vi "switch_data_process_switch-status.vi"() -> (0 "Switch_V_R":dbl[][](array[numeric]), 1 "Switch_V_L":dbl[][](array[numeric]), 2 "switch_FREQ_R":dbl[](array[numeric]), 3 "switch_FREQ_L":dbl[](array[numeric]), 4 "switch_RPF":dbl[](array[numeric]), 5 "switch_APF":dbl[](array[numeric]), 6 "switch_status":bool[](array[boolean]))   [LabVIEW 2016]
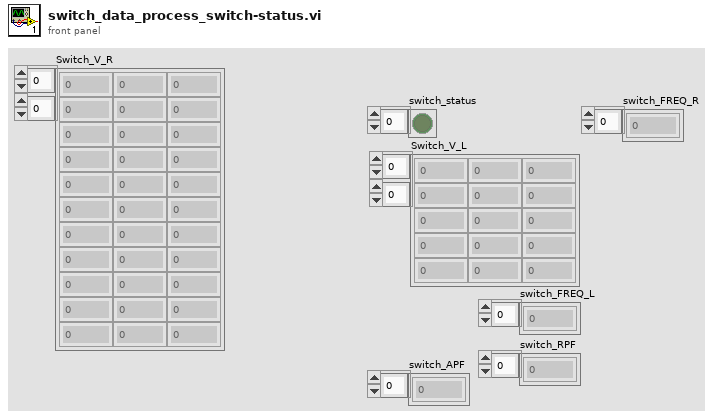
[diagram p1: front panel]
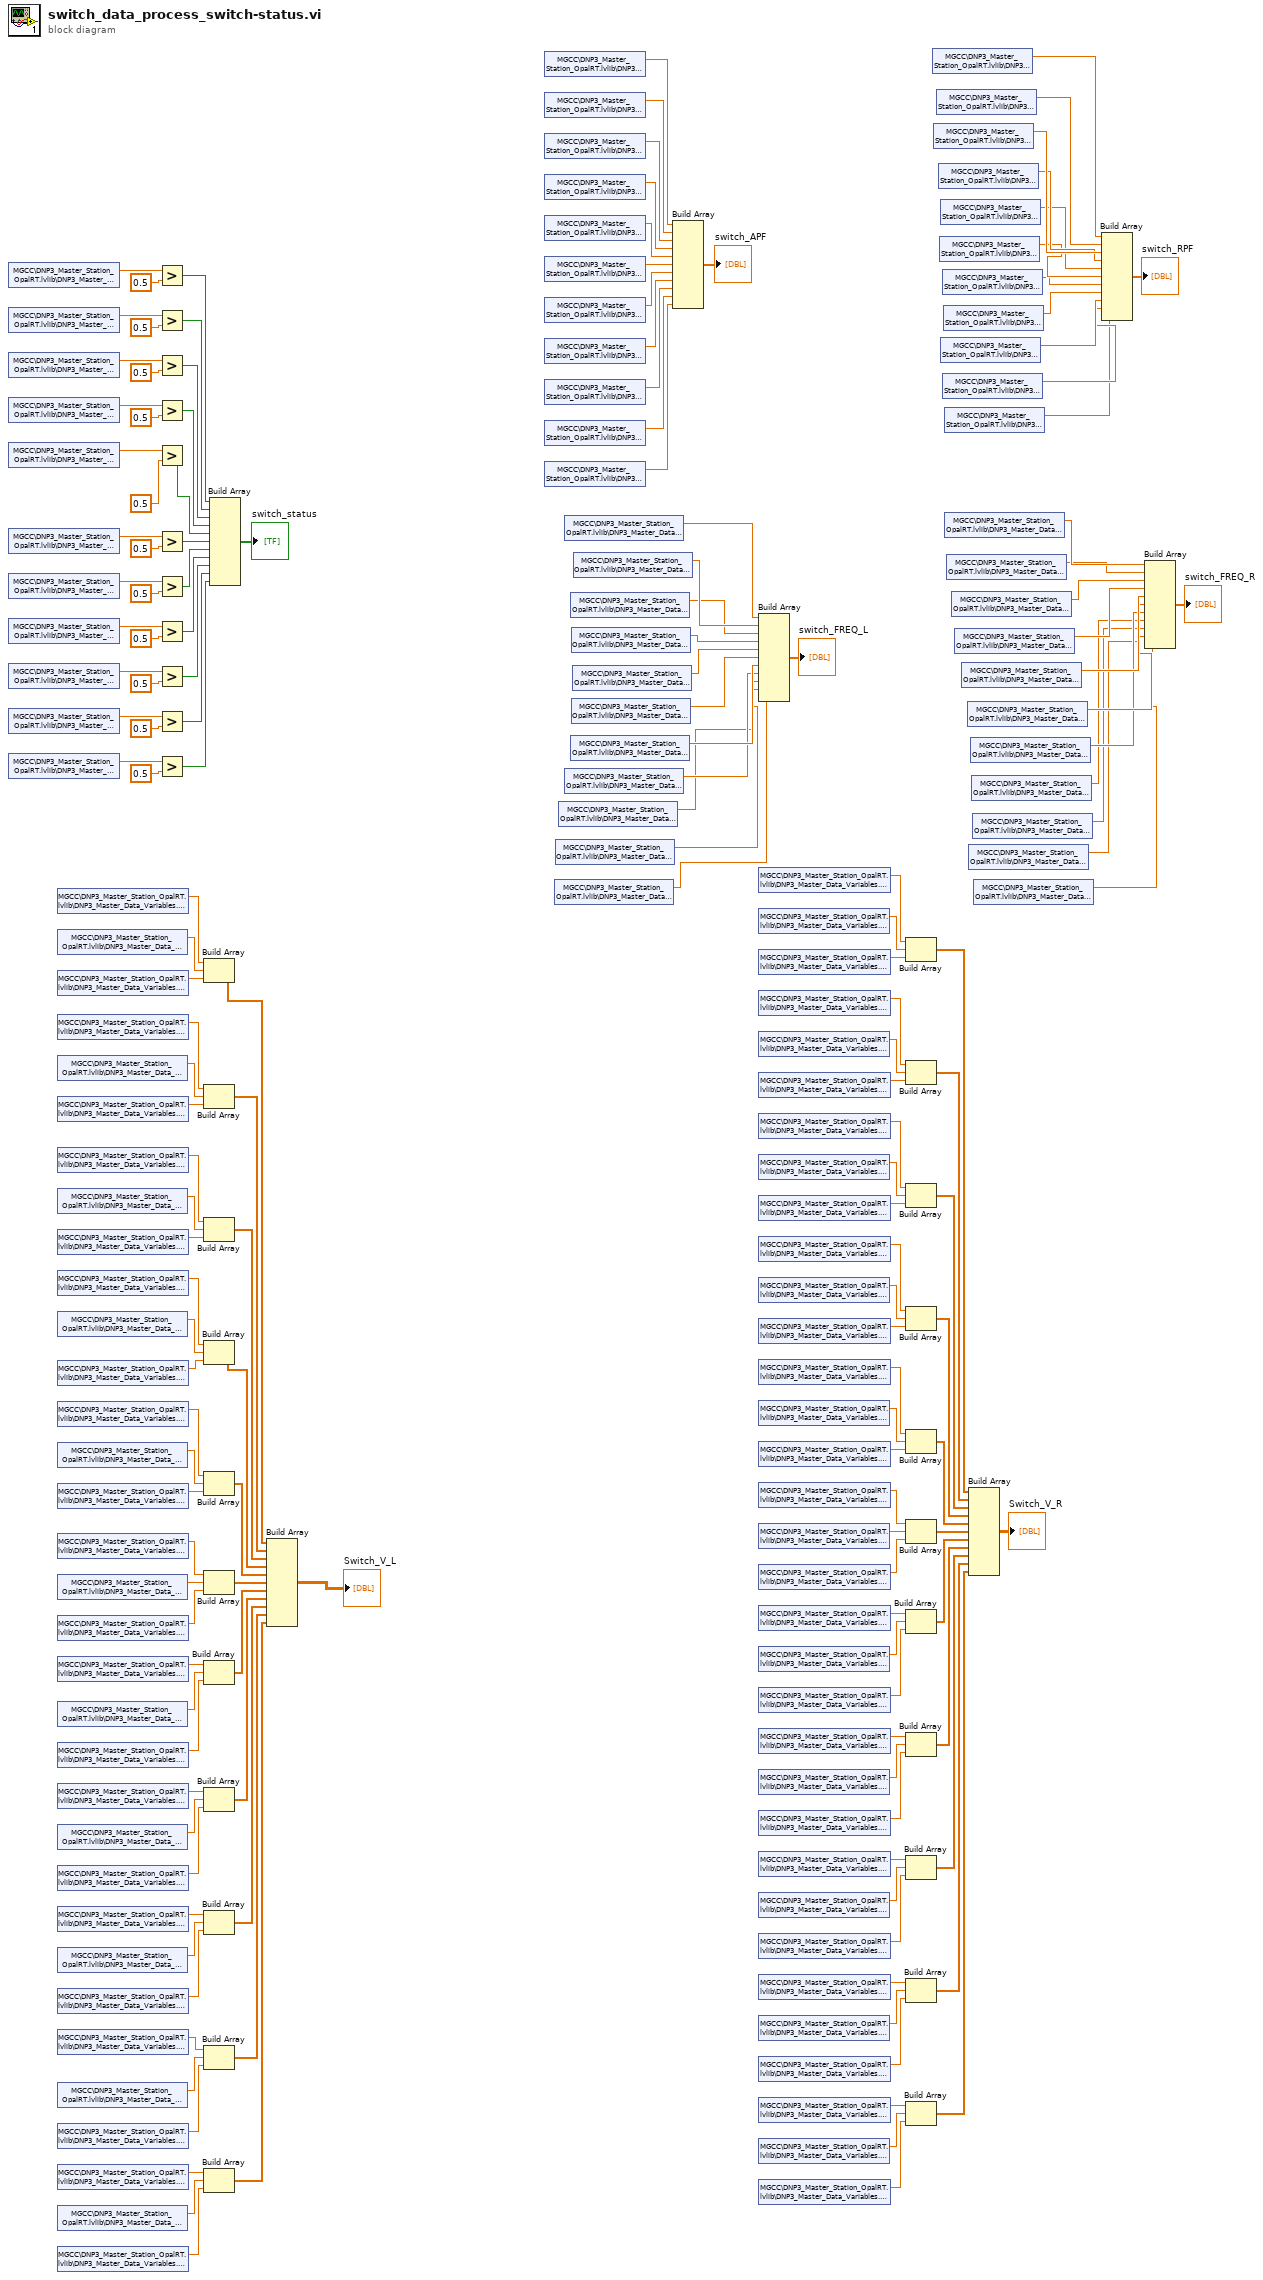
[diagram p0: block diagram]
diagram:
  n1 = shared-variable "MGCC\\DNP3_Master_Station_OpalRT.lvlib\\DNP3_Master_Data_Variables.lvlib\\MS_Analog_Status.lvlib\\S0102-status"() -> (w170:dbl)  [unwired: 1 in, 1 out]
  n2 = shared-variable "MGCC\\DNP3_Master_Station_OpalRT.lvlib\\DNP3_Master_Data_Variables.lvlib\\MS_Analog_Status.lvlib\\S0203-status"() -> (w159:dbl)  [unwired: 1 in, 1 out]
  n3 = shared-variable "MGCC\\DNP3_Master_Station_OpalRT.lvlib\\DNP3_Master_Data_Variables.lvlib\\MS_Analog_Status.lvlib\\S0304-status"() -> (w158:dbl)  [unwired: 1 in, 1 out]
  n4 = shared-variable "MGCC\\DNP3_Master_Station_OpalRT.lvlib\\DNP3_Master_Data_Variables.lvlib\\MS_Analog_Status.lvlib\\S0307-status"() -> (w157:dbl)  [unwired: 1 in, 1 out]
  n5 = shared-variable "MGCC\\DNP3_Master_Station_OpalRT.lvlib\\DNP3_Master_Data_Variables.lvlib\\MS_Analog_Status.lvlib\\S0405-status"() -> (w156:dbl)  [unwired: 1 in, 1 out]
  n6 = shared-variable "MGCC\\DNP3_Master_Station_OpalRT.lvlib\\DNP3_Master_Data_Variables.lvlib\\MS_Analog_Status.lvlib\\S0406-status"() -> (w155:dbl)  [unwired: 1 in, 1 out]
  n7 = shared-variable "MGCC\\DNP3_Master_Station_OpalRT.lvlib\\DNP3_Master_Data_Variables.lvlib\\MS_Analog_Status.lvlib\\S0708-status"() -> (w154:dbl)  [unwired: 1 in, 1 out]
  n8 = shared-variable "MGCC\\DNP3_Master_Station_OpalRT.lvlib\\DNP3_Master_Data_Variables.lvlib\\MS_Analog_Status.lvlib\\S0709-status"() -> (w153:dbl)  [unwired: 1 in, 1 out]
  n9 = shared-variable "MGCC\\DNP3_Master_Station_OpalRT.lvlib\\DNP3_Master_Data_Variables.lvlib\\MS_Analog_Status.lvlib\\S0910-status"() -> (w152:dbl)  [unwired: 1 in, 1 out]
  n10 = shared-variable "MGCC\\DNP3_Master_Station_OpalRT.lvlib\\DNP3_Master_Data_Variables.lvlib\\MS_Analog_Status.lvlib\\S1011-status"() -> (w151:dbl)  [unwired: 1 in, 1 out]
  n11 = shared-variable "MGCC\\DNP3_Master_Station_OpalRT.lvlib\\DNP3_Master_Data_Variables.lvlib\\MS_Analog_Status.lvlib\\S1114-status"() -> (w150:dbl)  [unwired: 1 in, 1 out]
  n12 = shared-variable "MGCC\\DNP3_Master_Station_OpalRT.lvlib\\DNP3_Master_Data_Variables.lvlib\\MS_Analog_Status.lvlib\\S0102-MAG-A-L"() -> (w138:dbl)  [unwired: 1 in, 1 out]
  n13 = shared-variable "MGCC\\DNP3_Master_Station_OpalRT.lvlib\\DNP3_Master_Data_Variables.lvlib\\MS_Analog_Status.lvlib\\S0102-MAG-B-L"() -> (w137:dbl)  [unwired: 1 in, 1 out]
  n14 = shared-variable "MGCC\\DNP3_Master_Station_OpalRT.lvlib\\DNP3_Master_Data_Variables.lvlib\\MS_Analog_Status.lvlib\\S0102-MAG-C-L"() -> (w136:dbl)  [unwired: 1 in, 1 out]
  n15 = shared-variable "MGCC\\DNP3_Master_Station_OpalRT.lvlib\\DNP3_Master_Data_Variables.lvlib\\MS_Analog_Status.lvlib\\S0203-MAG-A-L"() -> (w127:dbl)  [unwired: 1 in, 1 out]
  n16 = shared-variable "MGCC\\DNP3_Master_Station_OpalRT.lvlib\\DNP3_Master_Data_Variables.lvlib\\MS_Analog_Status.lvlib\\S0203-MAG-B-L"() -> (w126:dbl)  [unwired: 1 in, 1 out]
  n17 = shared-variable "MGCC\\DNP3_Master_Station_OpalRT.lvlib\\DNP3_Master_Data_Variables.lvlib\\MS_Analog_Status.lvlib\\S0203-MAG-C-L"() -> (w125:dbl)  [unwired: 1 in, 1 out]
  n18 = shared-variable "MGCC\\DNP3_Master_Station_OpalRT.lvlib\\DNP3_Master_Data_Variables.lvlib\\MS_Analog_Status.lvlib\\S0304-MAG-A-L"() -> (w122:dbl)  [unwired: 1 in, 1 out]
  n19 = shared-variable "MGCC\\DNP3_Master_Station_OpalRT.lvlib\\DNP3_Master_Data_Variables.lvlib\\MS_Analog_Status.lvlib\\S0304-MAG-B-L"() -> (w121:dbl)  [unwired: 1 in, 1 out]
  n20 = shared-variable "MGCC\\DNP3_Master_Station_OpalRT.lvlib\\DNP3_Master_Data_Variables.lvlib\\MS_Analog_Status.lvlib\\S0304-MAG-C-L"() -> (w120:dbl)  [unwired: 1 in, 1 out]
  n21 = shared-variable "MGCC\\DNP3_Master_Station_OpalRT.lvlib\\DNP3_Master_Data_Variables.lvlib\\MS_Analog_Status.lvlib\\S0307-MAG-A-L"() -> (w118:dbl)  [unwired: 1 in, 1 out]
  n22 = shared-variable "MGCC\\DNP3_Master_Station_OpalRT.lvlib\\DNP3_Master_Data_Variables.lvlib\\MS_Analog_Status.lvlib\\S0307-MAG-B-L"() -> (w117:dbl)  [unwired: 1 in, 1 out]
  n23 = shared-variable "MGCC\\DNP3_Master_Station_OpalRT.lvlib\\DNP3_Master_Data_Variables.lvlib\\MS_Analog_Status.lvlib\\S0307-MAG-C-L"() -> (w116:dbl)  [unwired: 1 in, 1 out]
  n24 = shared-variable "MGCC\\DNP3_Master_Station_OpalRT.lvlib\\DNP3_Master_Data_Variables.lvlib\\MS_Analog_Status.lvlib\\S0405-MAG-A-L"() -> (w114:dbl)  [unwired: 1 in, 1 out]
  n25 = shared-variable "MGCC\\DNP3_Master_Station_OpalRT.lvlib\\DNP3_Master_Data_Variables.lvlib\\MS_Analog_Status.lvlib\\S0405-MAG-B-L"() -> (w113:dbl)  [unwired: 1 in, 1 out]
  n26 = shared-variable "MGCC\\DNP3_Master_Station_OpalRT.lvlib\\DNP3_Master_Data_Variables.lvlib\\MS_Analog_Status.lvlib\\S0405-MAG-C-L"() -> (w112:dbl)  [unwired: 1 in, 1 out]
  n27 = shared-variable "MGCC\\DNP3_Master_Station_OpalRT.lvlib\\DNP3_Master_Data_Variables.lvlib\\MS_Analog_Status.lvlib\\S0406-MAG-A-L"() -> (w110:dbl)  [unwired: 1 in, 1 out]
  n28 = shared-variable "MGCC\\DNP3_Master_Station_OpalRT.lvlib\\DNP3_Master_Data_Variables.lvlib\\MS_Analog_Status.lvlib\\S0406-MAG-B-L"() -> (w109:dbl)  [unwired: 1 in, 1 out]
  n29 = shared-variable "MGCC\\DNP3_Master_Station_OpalRT.lvlib\\DNP3_Master_Data_Variables.lvlib\\MS_Analog_Status.lvlib\\S0406-MAG-C-L"() -> (w108:dbl)  [unwired: 1 in, 1 out]
  n30 = shared-variable "MGCC\\DNP3_Master_Station_OpalRT.lvlib\\DNP3_Master_Data_Variables.lvlib\\MS_Analog_Status.lvlib\\S0708-MAG-A-L"() -> (w106:dbl)  [unwired: 1 in, 1 out]
  n31 = shared-variable "MGCC\\DNP3_Master_Station_OpalRT.lvlib\\DNP3_Master_Data_Variables.lvlib\\MS_Analog_Status.lvlib\\S0708-MAG-B-L"() -> (w105:dbl)  [unwired: 1 in, 1 out]
  n32 = shared-variable "MGCC\\DNP3_Master_Station_OpalRT.lvlib\\DNP3_Master_Data_Variables.lvlib\\MS_Analog_Status.lvlib\\S0708-MAG-C-L"() -> (w104:dbl)  [unwired: 1 in, 1 out]
  n33 = shared-variable "MGCC\\DNP3_Master_Station_OpalRT.lvlib\\DNP3_Master_Data_Variables.lvlib\\MS_Analog_Status.lvlib\\S0709-MAG-A-L"() -> (w102:dbl)  [unwired: 1 in, 1 out]
  n34 = shared-variable "MGCC\\DNP3_Master_Station_OpalRT.lvlib\\DNP3_Master_Data_Variables.lvlib\\MS_Analog_Status.lvlib\\S0709-MAG-B-L"() -> (w101:dbl)  [unwired: 1 in, 1 out]
  n35 = shared-variable "MGCC\\DNP3_Master_Station_OpalRT.lvlib\\DNP3_Master_Data_Variables.lvlib\\MS_Analog_Status.lvlib\\S0709-MAG-C-L"() -> (w100:dbl)  [unwired: 1 in, 1 out]
  n36 = shared-variable "MGCC\\DNP3_Master_Station_OpalRT.lvlib\\DNP3_Master_Data_Variables.lvlib\\MS_Analog_Status.lvlib\\S0910-MAG-A-L"() -> (w98:dbl)  [unwired: 1 in, 1 out]
  n37 = shared-variable "MGCC\\DNP3_Master_Station_OpalRT.lvlib\\DNP3_Master_Data_Variables.lvlib\\MS_Analog_Status.lvlib\\S0910-MAG-B-L"() -> (w97:dbl)  [unwired: 1 in, 1 out]
  n38 = shared-variable "MGCC\\DNP3_Master_Station_OpalRT.lvlib\\DNP3_Master_Data_Variables.lvlib\\MS_Analog_Status.lvlib\\S0910-MAG-C-L"() -> (w96:dbl)  [unwired: 1 in, 1 out]
  n39 = shared-variable "MGCC\\DNP3_Master_Station_OpalRT.lvlib\\DNP3_Master_Data_Variables.lvlib\\MS_Analog_Status.lvlib\\S1011-MAG-A-L"() -> (w94:dbl)  [unwired: 1 in, 1 out]
  n40 = shared-variable "MGCC\\DNP3_Master_Station_OpalRT.lvlib\\DNP3_Master_Data_Variables.lvlib\\MS_Analog_Status.lvlib\\S1011-MAG-B-L"() -> (w93:dbl)  [unwired: 1 in, 1 out]
  n41 = shared-variable "MGCC\\DNP3_Master_Station_OpalRT.lvlib\\DNP3_Master_Data_Variables.lvlib\\MS_Analog_Status.lvlib\\S1011-MAG-C-L"() -> (w92:dbl)  [unwired: 1 in, 1 out]
  n42 = shared-variable "MGCC\\DNP3_Master_Station_OpalRT.lvlib\\DNP3_Master_Data_Variables.lvlib\\MS_Analog_Status.lvlib\\S1114-MAG-A-L"() -> (w90:dbl)  [unwired: 1 in, 1 out]
  n43 = shared-variable "MGCC\\DNP3_Master_Station_OpalRT.lvlib\\DNP3_Master_Data_Variables.lvlib\\MS_Analog_Status.lvlib\\S1114-MAG-B-L"() -> (w89:dbl)  [unwired: 1 in, 1 out]
  n44 = shared-variable "MGCC\\DNP3_Master_Station_OpalRT.lvlib\\DNP3_Master_Data_Variables.lvlib\\MS_Analog_Status.lvlib\\S1114-MAG-C-L"() -> (w88:dbl)  [unwired: 1 in, 1 out]
  n45 = Greater?(x=w170, y=0.5) -> (0:w171:bool)
  n46 = Greater?(x=w159, y=0.5) -> (0:w149:bool)
  n47 = Greater?(x=w158, y=0.5) -> (0:w148:bool)
  n48 = Greater?(x=w157, y=0.5) -> (0:w147:bool)
  n49 = Greater?(x=w156, y=0.5) -> (0:w146:bool)
  n50 = Greater?(x=w155, y=0.5) -> (0:w145:bool)
  n51 = Greater?(x=w154, y=0.5) -> (0:w144:bool)
  n52 = Greater?(x=w153, y=0.5) -> (0:w143:bool)
  n53 = Greater?(x=w152, y=0.5) -> (0:w142:bool)
  n54 = Greater?(x=w151, y=0.5) -> (0:w141:bool)
  n55 = Greater?(x=w150, y=0.5) -> (0:w140:bool)
  n56 = Build Array(w138, w137, w136) -> (w135:dbl[])
  n57 = Build Array(w127, w126, w125) -> (w124:dbl[])
  n58 = Build Array(w122, w121, w120) -> (w119:dbl[])
  n59 = Build Array(w118, w117, w116) -> (w115:dbl[])
  n60 = Build Array(w114, w113, w112) -> (w111:dbl[])
  n61 = Build Array(w110, w109, w108) -> (w107:dbl[])
  n62 = Build Array(w106, w105, w104) -> (w103:dbl[])
  n63 = Build Array(w102, w101, w100) -> (w99:dbl[])
  n64 = Build Array(w98, w97, w96) -> (w95:dbl[])
  n65 = Build Array(w94, w93, w92) -> (w91:dbl[])
  n66 = Build Array(w90, w89, w88) -> (w87:dbl[])
  n67 = Build Array(w171, w149, w148, w147, w146, w145, w144, w143, w142, w141, w140) -> (→"switch_status":bool[])
  n68 = Build Array(w135, w124, w119, w115, w111, w107, w103, w99, w95, w91, w87) -> (→"Switch_V_L":dbl[][])
  n69 = shared-variable "MGCC\\DNP3_Master_Station_OpalRT.lvlib\\DNP3_Master_Data_Variables.lvlib\\MS_Analog_Status.lvlib\\S0102-APF"() -> (w48:dbl)  [unwired: 1 in, 1 out]
  n70 = shared-variable "MGCC\\DNP3_Master_Station_OpalRT.lvlib\\DNP3_Master_Data_Variables.lvlib\\MS_Analog_Status.lvlib\\S0203-APF"() -> (w47:dbl)  [unwired: 1 in, 1 out]
  n71 = shared-variable "MGCC\\DNP3_Master_Station_OpalRT.lvlib\\DNP3_Master_Data_Variables.lvlib\\MS_Analog_Status.lvlib\\S0304-APF"() -> (w46:dbl)  [unwired: 1 in, 1 out]
  n72 = shared-variable "MGCC\\DNP3_Master_Station_OpalRT.lvlib\\DNP3_Master_Data_Variables.lvlib\\MS_Analog_Status.lvlib\\S0307-APF"() -> (w45:dbl)  [unwired: 1 in, 1 out]
  n73 = shared-variable "MGCC\\DNP3_Master_Station_OpalRT.lvlib\\DNP3_Master_Data_Variables.lvlib\\MS_Analog_Status.lvlib\\S0405-APF"() -> (w44:dbl)  [unwired: 1 in, 1 out]
  n74 = shared-variable "MGCC\\DNP3_Master_Station_OpalRT.lvlib\\DNP3_Master_Data_Variables.lvlib\\MS_Analog_Status.lvlib\\S0406-APF"() -> (w43:dbl)  [unwired: 1 in, 1 out]
  n75 = shared-variable "MGCC\\DNP3_Master_Station_OpalRT.lvlib\\DNP3_Master_Data_Variables.lvlib\\MS_Analog_Status.lvlib\\S0708-APF"() -> (w42:dbl)  [unwired: 1 in, 1 out]
  n76 = shared-variable "MGCC\\DNP3_Master_Station_OpalRT.lvlib\\DNP3_Master_Data_Variables.lvlib\\MS_Analog_Status.lvlib\\S0709-APF"() -> (w41:dbl)  [unwired: 1 in, 1 out]
  n77 = shared-variable "MGCC\\DNP3_Master_Station_OpalRT.lvlib\\DNP3_Master_Data_Variables.lvlib\\MS_Analog_Status.lvlib\\S0910-APF"() -> (w40:dbl)  [unwired: 1 in, 1 out]
  n78 = shared-variable "MGCC\\DNP3_Master_Station_OpalRT.lvlib\\DNP3_Master_Data_Variables.lvlib\\MS_Analog_Status.lvlib\\S1011-APF"() -> (w39:dbl)  [unwired: 1 in, 1 out]
  n79 = shared-variable "MGCC\\DNP3_Master_Station_OpalRT.lvlib\\DNP3_Master_Data_Variables.lvlib\\MS_Analog_Status.lvlib\\S1114-APF"() -> (w38:dbl)  [unwired: 1 in, 1 out]
  n80 = shared-variable "MGCC\\DNP3_Master_Station_OpalRT.lvlib\\DNP3_Master_Data_Variables.lvlib\\MS_Analog_Status.lvlib\\S1114-FREQ-L"() -> (w26:dbl)  [unwired: 1 in, 1 out]
  n81 = shared-variable "MGCC\\DNP3_Master_Station_OpalRT.lvlib\\DNP3_Master_Data_Variables.lvlib\\MS_Analog_Status.lvlib\\S1011-FREQ-L"() -> (w27:dbl)  [unwired: 1 in, 1 out]
  n82 = shared-variable "MGCC\\DNP3_Master_Station_OpalRT.lvlib\\DNP3_Master_Data_Variables.lvlib\\MS_Analog_Status.lvlib\\S0910-FREQ-L"() -> (w28:dbl)  [unwired: 1 in, 1 out]
  n83 = shared-variable "MGCC\\DNP3_Master_Station_OpalRT.lvlib\\DNP3_Master_Data_Variables.lvlib\\MS_Analog_Status.lvlib\\S0102-FREQ-L"() -> (w36:dbl)  [unwired: 1 in, 1 out]
  n84 = shared-variable "MGCC\\DNP3_Master_Station_OpalRT.lvlib\\DNP3_Master_Data_Variables.lvlib\\MS_Analog_Status.lvlib\\S0709-FREQ-L"() -> (w29:dbl)  [unwired: 1 in, 1 out]
  n85 = shared-variable "MGCC\\DNP3_Master_Station_OpalRT.lvlib\\DNP3_Master_Data_Variables.lvlib\\MS_Analog_Status.lvlib\\S0304-FREQ-L"() -> (w34:dbl)  [unwired: 1 in, 1 out]
  n86 = shared-variable "MGCC\\DNP3_Master_Station_OpalRT.lvlib\\DNP3_Master_Data_Variables.lvlib\\MS_Analog_Status.lvlib\\S0708-FREQ-L"() -> (w30:dbl)  [unwired: 1 in, 1 out]
  n87 = shared-variable "MGCC\\DNP3_Master_Station_OpalRT.lvlib\\DNP3_Master_Data_Variables.lvlib\\MS_Analog_Status.lvlib\\S0307-FREQ-L"() -> (w33:dbl)  [unwired: 1 in, 1 out]
  n88 = shared-variable "MGCC\\DNP3_Master_Station_OpalRT.lvlib\\DNP3_Master_Data_Variables.lvlib\\MS_Analog_Status.lvlib\\S0406-FREQ-L"() -> (w31:dbl)  [unwired: 1 in, 1 out]
  n89 = shared-variable "MGCC\\DNP3_Master_Station_OpalRT.lvlib\\DNP3_Master_Data_Variables.lvlib\\MS_Analog_Status.lvlib\\S0405-FREQ-L"() -> (w32:dbl)  [unwired: 1 in, 1 out]
  n90 = shared-variable "MGCC\\DNP3_Master_Station_OpalRT.lvlib\\DNP3_Master_Data_Variables.lvlib\\MS_Analog_Status.lvlib\\S0203-FREQ-L"() -> (w35:dbl)  [unwired: 1 in, 1 out]
  n91 = Build Array(w48, w47, w46, w45, w44, w43, w42, w41, w40, w39, w38) -> (→"switch_APF":dbl[])
  n92 = Build Array(w36, w35, w34, w33, w32, w31, w30, w29, w28, w27, w26) -> (→"switch_FREQ_L":dbl[])
  n93 = shared-variable "MGCC\\DNP3_Master_Station_OpalRT.lvlib\\DNP3_Master_Data_Variables.lvlib\\MS_Analog_Status.lvlib\\S0102-MAG-A-R"() -> (w134:dbl)  [unwired: 1 in, 1 out]
  n94 = shared-variable "MGCC\\DNP3_Master_Station_OpalRT.lvlib\\DNP3_Master_Data_Variables.lvlib\\MS_Analog_Status.lvlib\\S0102-MAG-B-R"() -> (w133:dbl)  [unwired: 1 in, 1 out]
  n95 = shared-variable "MGCC\\DNP3_Master_Station_OpalRT.lvlib\\DNP3_Master_Data_Variables.lvlib\\MS_Analog_Status.lvlib\\S0102-MAG-C-R"() -> (w132:dbl)  [unwired: 1 in, 1 out]
  n96 = shared-variable "MGCC\\DNP3_Master_Station_OpalRT.lvlib\\DNP3_Master_Data_Variables.lvlib\\MS_Analog_Status.lvlib\\S0203-MAG-A-R"() -> (w130:dbl)  [unwired: 1 in, 1 out]
  n97 = shared-variable "MGCC\\DNP3_Master_Station_OpalRT.lvlib\\DNP3_Master_Data_Variables.lvlib\\MS_Analog_Status.lvlib\\S0203-MAG-B-R"() -> (w129:dbl)  [unwired: 1 in, 1 out]
  n98 = shared-variable "MGCC\\DNP3_Master_Station_OpalRT.lvlib\\DNP3_Master_Data_Variables.lvlib\\MS_Analog_Status.lvlib\\S0203-MAG-C-R"() -> (w128:dbl)  [unwired: 1 in, 1 out]
  n99 = shared-variable "MGCC\\DNP3_Master_Station_OpalRT.lvlib\\DNP3_Master_Data_Variables.lvlib\\MS_Analog_Status.lvlib\\S0304-MAG-A-R"() -> (w86:dbl)  [unwired: 1 in, 1 out]
  n100 = shared-variable "MGCC\\DNP3_Master_Station_OpalRT.lvlib\\DNP3_Master_Data_Variables.lvlib\\MS_Analog_Status.lvlib\\S0304-MAG-B-R"() -> (w85:dbl)  [unwired: 1 in, 1 out]
  n101 = shared-variable "MGCC\\DNP3_Master_Station_OpalRT.lvlib\\DNP3_Master_Data_Variables.lvlib\\MS_Analog_Status.lvlib\\S0304-MAG-C-R"() -> (w84:dbl)  [unwired: 1 in, 1 out]
  n102 = shared-variable "MGCC\\DNP3_Master_Station_OpalRT.lvlib\\DNP3_Master_Data_Variables.lvlib\\MS_Analog_Status.lvlib\\S0307-MAG-A-R"() -> (w82:dbl)  [unwired: 1 in, 1 out]
  n103 = shared-variable "MGCC\\DNP3_Master_Station_OpalRT.lvlib\\DNP3_Master_Data_Variables.lvlib\\MS_Analog_Status.lvlib\\S0307-MAG-B-R"() -> (w81:dbl)  [unwired: 1 in, 1 out]
  n104 = shared-variable "MGCC\\DNP3_Master_Station_OpalRT.lvlib\\DNP3_Master_Data_Variables.lvlib\\MS_Analog_Status.lvlib\\S0307-MAG-C-R"() -> (w80:dbl)  [unwired: 1 in, 1 out]
  n105 = shared-variable "MGCC\\DNP3_Master_Station_OpalRT.lvlib\\DNP3_Master_Data_Variables.lvlib\\MS_Analog_Status.lvlib\\S0405-MAG-A-R"() -> (w78:dbl)  [unwired: 1 in, 1 out]
  n106 = shared-variable "MGCC\\DNP3_Master_Station_OpalRT.lvlib\\DNP3_Master_Data_Variables.lvlib\\MS_Analog_Status.lvlib\\S0405-MAG-B-R"() -> (w77:dbl)  [unwired: 1 in, 1 out]
  n107 = shared-variable "MGCC\\DNP3_Master_Station_OpalRT.lvlib\\DNP3_Master_Data_Variables.lvlib\\MS_Analog_Status.lvlib\\S0405-MAG-C-R"() -> (w76:dbl)  [unwired: 1 in, 1 out]
  n108 = shared-variable "MGCC\\DNP3_Master_Station_OpalRT.lvlib\\DNP3_Master_Data_Variables.lvlib\\MS_Analog_Status.lvlib\\S0406-MAG-A-R"() -> (w74:dbl)  [unwired: 1 in, 1 out]
  n109 = shared-variable "MGCC\\DNP3_Master_Station_OpalRT.lvlib\\DNP3_Master_Data_Variables.lvlib\\MS_Analog_Status.lvlib\\S0406-MAG-B-R"() -> (w73:dbl)  [unwired: 1 in, 1 out]
  n110 = shared-variable "MGCC\\DNP3_Master_Station_OpalRT.lvlib\\DNP3_Master_Data_Variables.lvlib\\MS_Analog_Status.lvlib\\S0406-MAG-C-R"() -> (w72:dbl)  [unwired: 1 in, 1 out]
  n111 = shared-variable "MGCC\\DNP3_Master_Station_OpalRT.lvlib\\DNP3_Master_Data_Variables.lvlib\\MS_Analog_Status.lvlib\\S0708-MAG-A-R"() -> (w70:dbl)  [unwired: 1 in, 1 out]
  n112 = shared-variable "MGCC\\DNP3_Master_Station_OpalRT.lvlib\\DNP3_Master_Data_Variables.lvlib\\MS_Analog_Status.lvlib\\S0708-MAG-B-R"() -> (w69:dbl)  [unwired: 1 in, 1 out]
  n113 = shared-variable "MGCC\\DNP3_Master_Station_OpalRT.lvlib\\DNP3_Master_Data_Variables.lvlib\\MS_Analog_Status.lvlib\\S0708-MAG-C-R"() -> (w68:dbl)  [unwired: 1 in, 1 out]
  n114 = shared-variable "MGCC\\DNP3_Master_Station_OpalRT.lvlib\\DNP3_Master_Data_Variables.lvlib\\MS_Analog_Status.lvlib\\S0709-MAG-A-R"() -> (w66:dbl)  [unwired: 1 in, 1 out]
  n115 = shared-variable "MGCC\\DNP3_Master_Station_OpalRT.lvlib\\DNP3_Master_Data_Variables.lvlib\\MS_Analog_Status.lvlib\\S0709-MAG-B-R"() -> (w65:dbl)  [unwired: 1 in, 1 out]
  n116 = shared-variable "MGCC\\DNP3_Master_Station_OpalRT.lvlib\\DNP3_Master_Data_Variables.lvlib\\MS_Analog_Status.lvlib\\S0709-MAG-C-R"() -> (w64:dbl)  [unwired: 1 in, 1 out]
  n117 = shared-variable "MGCC\\DNP3_Master_Station_OpalRT.lvlib\\DNP3_Master_Data_Variables.lvlib\\MS_Analog_Status.lvlib\\S0910-MAG-A-R"() -> (w62:dbl)  [unwired: 1 in, 1 out]
  n118 = shared-variable "MGCC\\DNP3_Master_Station_OpalRT.lvlib\\DNP3_Master_Data_Variables.lvlib\\MS_Analog_Status.lvlib\\S0910-MAG-B-R"() -> (w61:dbl)  [unwired: 1 in, 1 out]
  n119 = shared-variable "MGCC\\DNP3_Master_Station_OpalRT.lvlib\\DNP3_Master_Data_Variables.lvlib\\MS_Analog_Status.lvlib\\S0910-MAG-C-R"() -> (w60:dbl)  [unwired: 1 in, 1 out]
  n120 = shared-variable "MGCC\\DNP3_Master_Station_OpalRT.lvlib\\DNP3_Master_Data_Variables.lvlib\\MS_Analog_Status.lvlib\\S1011-MAG-A-R"() -> (w58:dbl)  [unwired: 1 in, 1 out]
  n121 = shared-variable "MGCC\\DNP3_Master_Station_OpalRT.lvlib\\DNP3_Master_Data_Variables.lvlib\\MS_Analog_Status.lvlib\\S1011-MAG-B-R"() -> (w57:dbl)  [unwired: 1 in, 1 out]
  n122 = shared-variable "MGCC\\DNP3_Master_Station_OpalRT.lvlib\\DNP3_Master_Data_Variables.lvlib\\MS_Analog_Status.lvlib\\S1011-MAG-C-R"() -> (w56:dbl)  [unwired: 1 in, 1 out]
  n123 = shared-variable "MGCC\\DNP3_Master_Station_OpalRT.lvlib\\DNP3_Master_Data_Variables.lvlib\\MS_Analog_Status.lvlib\\S1114-MAG-A-R"() -> (w54:dbl)  [unwired: 1 in, 1 out]
  n124 = shared-variable "MGCC\\DNP3_Master_Station_OpalRT.lvlib\\DNP3_Master_Data_Variables.lvlib\\MS_Analog_Status.lvlib\\S1114-MAG-B-R"() -> (w53:dbl)  [unwired: 1 in, 1 out]
  n125 = shared-variable "MGCC\\DNP3_Master_Station_OpalRT.lvlib\\DNP3_Master_Data_Variables.lvlib\\MS_Analog_Status.lvlib\\S1114-MAG-C-R"() -> (w52:dbl)  [unwired: 1 in, 1 out]
  n126 = Build Array(w134, w133, w132) -> (w131:dbl[])
  n127 = Build Array(w130, w129, w128) -> (w123:dbl[])
  n128 = Build Array(w86, w85, w84) -> (w83:dbl[])
  n129 = Build Array(w82, w81, w80) -> (w79:dbl[])
  n130 = Build Array(w78, w77, w76) -> (w75:dbl[])
  n131 = Build Array(w74, w73, w72) -> (w71:dbl[])
  n132 = Build Array(w70, w69, w68) -> (w67:dbl[])
  n133 = Build Array(w66, w65, w64) -> (w63:dbl[])
  n134 = Build Array(w62, w61, w60) -> (w59:dbl[])
  n135 = Build Array(w58, w57, w56) -> (w55:dbl[])
  n136 = Build Array(w54, w53, w52) -> (w51:dbl[])
  n137 = shared-variable "MGCC\\DNP3_Master_Station_OpalRT.lvlib\\DNP3_Master_Data_Variables.lvlib\\MS_Analog_Status.lvlib\\S0102-RPF"() -> (w24:dbl)  [unwired: 1 in, 1 out]
  n138 = shared-variable "MGCC\\DNP3_Master_Station_OpalRT.lvlib\\DNP3_Master_Data_Variables.lvlib\\MS_Analog_Status.lvlib\\S0304-RPF"() -> (w22:dbl)  [unwired: 1 in, 1 out]
  n139 = shared-variable "MGCC\\DNP3_Master_Station_OpalRT.lvlib\\DNP3_Master_Data_Variables.lvlib\\MS_Analog_Status.lvlib\\S0203-RPF"() -> (w23:dbl)  [unwired: 1 in, 1 out]
  n140 = shared-variable "MGCC\\DNP3_Master_Station_OpalRT.lvlib\\DNP3_Master_Data_Variables.lvlib\\MS_Analog_Status.lvlib\\S0307-RPF"() -> (w21:dbl)  [unwired: 1 in, 1 out]
  n141 = shared-variable "MGCC\\DNP3_Master_Station_OpalRT.lvlib\\DNP3_Master_Data_Variables.lvlib\\MS_Analog_Status.lvlib\\S0406-RPF"() -> (w19:dbl)  [unwired: 1 in, 1 out]
  n142 = shared-variable "MGCC\\DNP3_Master_Station_OpalRT.lvlib\\DNP3_Master_Data_Variables.lvlib\\MS_Analog_Status.lvlib\\S0405-RPF"() -> (w20:dbl)  [unwired: 1 in, 1 out]
  n143 = shared-variable "MGCC\\DNP3_Master_Station_OpalRT.lvlib\\DNP3_Master_Data_Variables.lvlib\\MS_Analog_Status.lvlib\\S0910-RPF"() -> (w16:dbl)  [unwired: 1 in, 1 out]
  n144 = shared-variable "MGCC\\DNP3_Master_Station_OpalRT.lvlib\\DNP3_Master_Data_Variables.lvlib\\MS_Analog_Status.lvlib\\S0708-RPF"() -> (w18:dbl)  [unwired: 1 in, 1 out]
  n145 = shared-variable "MGCC\\DNP3_Master_Station_OpalRT.lvlib\\DNP3_Master_Data_Variables.lvlib\\MS_Analog_Status.lvlib\\S1011-RPF"() -> (w15:dbl)  [unwired: 1 in, 1 out]
  n146 = shared-variable "MGCC\\DNP3_Master_Station_OpalRT.lvlib\\DNP3_Master_Data_Variables.lvlib\\MS_Analog_Status.lvlib\\S0709-RPF"() -> (w17:dbl)  [unwired: 1 in, 1 out]
  n147 = shared-variable "MGCC\\DNP3_Master_Station_OpalRT.lvlib\\DNP3_Master_Data_Variables.lvlib\\MS_Analog_Status.lvlib\\S1114-RPF"() -> (w14:dbl)  [unwired: 1 in, 1 out]
  n148 = shared-variable "MGCC\\DNP3_Master_Station_OpalRT.lvlib\\DNP3_Master_Data_Variables.lvlib\\MS_Analog_Status.lvlib\\S0102-FREQ-R"() -> (w12:dbl)  [unwired: 1 in, 1 out]
  n149 = shared-variable "MGCC\\DNP3_Master_Station_OpalRT.lvlib\\DNP3_Master_Data_Variables.lvlib\\MS_Analog_Status.lvlib\\S0203-FREQ-R"() -> (w11:dbl)  [unwired: 1 in, 1 out]
  n150 = shared-variable "MGCC\\DNP3_Master_Station_OpalRT.lvlib\\DNP3_Master_Data_Variables.lvlib\\MS_Analog_Status.lvlib\\S0304-FREQ-R"() -> (w10:dbl)  [unwired: 1 in, 1 out]
  n151 = shared-variable "MGCC\\DNP3_Master_Station_OpalRT.lvlib\\DNP3_Master_Data_Variables.lvlib\\MS_Analog_Status.lvlib\\S0307-FREQ-R"() -> (w9:dbl)  [unwired: 1 in, 1 out]
  n152 = shared-variable "MGCC\\DNP3_Master_Station_OpalRT.lvlib\\DNP3_Master_Data_Variables.lvlib\\MS_Analog_Status.lvlib\\S0405-FREQ-R"() -> (w8:dbl)  [unwired: 1 in, 1 out]
  n153 = shared-variable "MGCC\\DNP3_Master_Station_OpalRT.lvlib\\DNP3_Master_Data_Variables.lvlib\\MS_Analog_Status.lvlib\\S0406-FREQ-R"() -> (w7:dbl)  [unwired: 1 in, 1 out]
  n154 = shared-variable "MGCC\\DNP3_Master_Station_OpalRT.lvlib\\DNP3_Master_Data_Variables.lvlib\\MS_Analog_Status.lvlib\\S1011-FREQ-R"() -> (w3:dbl)  [unwired: 1 in, 1 out]
  n155 = Build Array(w131, w123, w83, w79, w75, w71, w67, w63, w59, w55, w51) -> (→"Switch_V_R":dbl[][])
  n156 = shared-variable "MGCC\\DNP3_Master_Station_OpalRT.lvlib\\DNP3_Master_Data_Variables.lvlib\\MS_Analog_Status.lvlib\\S0708-FREQ-R"() -> (w6:dbl)  [unwired: 1 in, 1 out]
  n157 = shared-variable "MGCC\\DNP3_Master_Station_OpalRT.lvlib\\DNP3_Master_Data_Variables.lvlib\\MS_Analog_Status.lvlib\\S0709-FREQ-R"() -> (w5:dbl)  [unwired: 1 in, 1 out]
  n158 = shared-variable "MGCC\\DNP3_Master_Station_OpalRT.lvlib\\DNP3_Master_Data_Variables.lvlib\\MS_Analog_Status.lvlib\\S0910-FREQ-R"() -> (w4:dbl)  [unwired: 1 in, 1 out]
  n159 = shared-variable "MGCC\\DNP3_Master_Station_OpalRT.lvlib\\DNP3_Master_Data_Variables.lvlib\\MS_Analog_Status.lvlib\\S1114-FREQ-R"() -> (w2:dbl)  [unwired: 1 in, 1 out]
  n160 = Build Array(w24, w23, w22, w21, w20, w19, w18, w17, w16, w15, w14) -> (→"switch_RPF":dbl[])
  n161 = Build Array(w12, w11, w10, w9, w8, w7, w6, w5, w4, w3, w2) -> (→"switch_FREQ_R":dbl[])
